vi "List Folder.vi"(0 "stripped path":path, 1 "depth":i32=-1, 2 "ģʽ":string, 5 "error in (no error)":errorcluster, 7 "depth index":i32=1) -> (14 "files":path[](array[path]), 19 "error out":errorcluster)   [LabVIEW 2015]
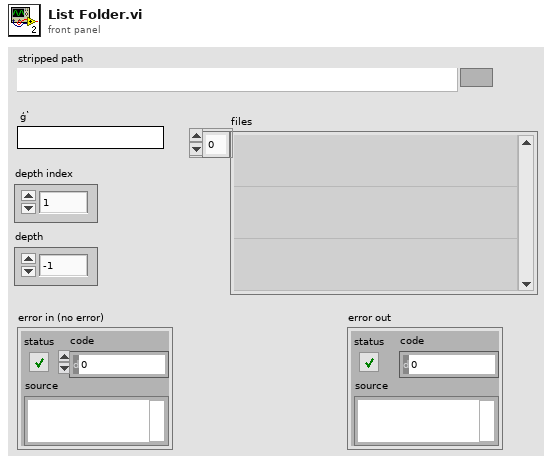
[diagram p1: front panel]
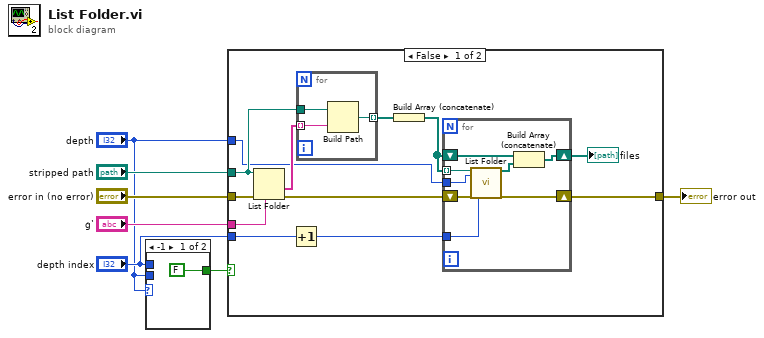
[diagram p0: block diagram]
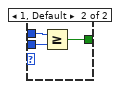
[diagram p2: hidden frame]
diagram:
  n1 = case shown="-1" "depth" {
    tunnel: "depth index" -> [_ w11]
    tunnel: "depth" -> [_ w10]
    tunnel: [FALSE w9] -> w4
    frame -1 {
    }
    frame 1, Default {
      n2 = Greater Or Equal?(x=w11, y=w10) -> (x >= y?=w9:bool)
    }
  }
  n3 = case shown="False" w4 {
    tunnel: "error in (no error)" -> [w23 w35]
    tunnel: "stripped path" -> [w22 _]
    tunnel: "depth index" -> [w16 _]
    tunnel: "depth" -> [w15 _]
    tunnel: [w14 w35] -> w3
    tunnel: "ģʽ" -> [w13 _]
    frame False {
      n4 = List Folder(path=w22, pattern=w13, error in=w23) -> (folder names=w20:string[], error out=w19:errorcluster)  [unwired: 1 in, 2 out]
      n5 = Increment(x=w16) -> (x+1=w17:i32)
      n6 = for {
        tunnel: w20 -> [w33] mode=indexing
        tunnel: w22 -> [w34]
        tunnel: [w32] -> w18 mode=indexing
        n7 = Build Path(base path=w34, name or relative path=w33) -> (appended path=w32:path)
      }
      n8 = Build Array (concatenate)(w18) -> (w12:path[])
      n9 = for {
        tunnel: w12 -> [w27] mode=indexing
        shift-right: [w30] -> w14
        shift-left: w19 -> [w31]
        shift-right: [w28] -> w21
        shift-left: w12 -> [w29]
        tunnel: w15 -> [w25]
        tunnel: w17 -> [w24]
        n10 = call "List Folder.vi"("stripped path"=w27, "depth"=w25, "error in (no error)"=w31, "depth index"=w24) -> ("files"=w26:path[], "error out"=w30:errorcluster)  [unwired: 14 in]
        n11 = Build Array (concatenate)(w29, w26) -> (w28:path[])
      }
      "files" <- w21
    }
    frame True {
    }
  }
  "error out" <- w3
